vi "Transfer Observer Resources.vi"(10 "Recipient Observer In":refnum<class "IObserver.lvclass">, 11 "Running Observer":refnum<class "IObserver.lvclass">) -> (2 "Recipient Observer Out":refnum<class "IObserver.lvclass">)   [LabVIEW 2017, in "IObserver.lvlib" / "IObserver.lvclass"]
uses:
  IObserver.lvclass
  IObserver.lvclass/IObserver.ctl
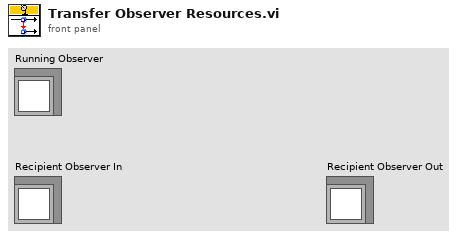
[diagram p1: front panel]
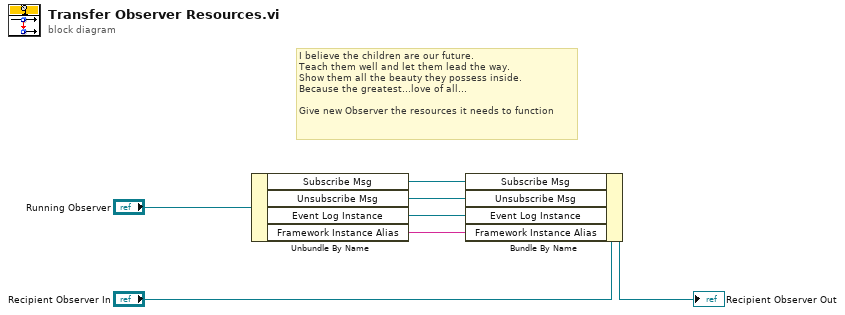
[diagram p0: block diagram]
diagram:
  # "I believe the children are our future.\nTeach them well and let them lead the way.\nShow them all the beauty they possess inside.\nBecause the greatest...love of all...\n\nGive new Observer the resources it needs to function"
  n1 = Unbundle By Name("Running Observer") -> ("Subscribe Msg"=w4:refnum<class "Subscribe Msg.lvclass">, "Unsubscribe Msg"=w3:refnum<class "Unsubscribe Msg.lvclass">, "Event Log Instance"=w2:refnum<class "LoggerReference.lvclass">, "Framework Instance Alias"=w1:string)
  n2 = Bundle By Name(cluster="Recipient Observer In", "Subscribe Msg"=w4, "Unsubscribe Msg"=w3, "Event Log Instance"=w2, "Framework Instance Alias"=w1) -> (→"Recipient Observer Out":refnum<class "IObserver.lvclass">)
